vi "main.vi"() -> ()   [LabVIEW 2016]
uses:
  <vilib>/Simulation/Scripting/Companion Diagram/SimConfigNode/SimDog.xnode
  <vilib>/Simulation/Implementation/Shared/SIMSCR Execution Mode.ctl
  <vilib>/Simulation/Scripting/Companion Diagram/SimConfigNode/_simSolvers.ctl
  <vilib>/Simulation/Scripting/Companion Diagram/SimConfigNode/SimParams.ctl
  <vilib>/Simulation/Implementation/XNodeFramework/SimXNode/SimX.xnode
  <vilib>/Simulation/Model Libraries/PID/SIM PID.vi
  <vilib>/Simulation/SignalArithmetic/Implementation/NILVSim Gain.llb/SIM Gain (scalar).vi
  <vilib>/Simulation/Utility/Implementation/SIM Halt.vi
  <vilib>/Simulation/ContinuousLinear/Implementation/NILVSim Integrator new.llb/SIM Integrator (scalar).vi
  <vilib>/Simulation/ContinuousLinear/Implementation/NILVSim Transfer Function.llb/SIM Transfer Function (SISO).vi
  <vilib>/Simulation/Model Libraries/PID/SIM PID (Parallel).vi
  <vilib>/Instr/_visa.llb/VISA Configure Serial Port (Instr).vi
panel:
  in  "lower limit":dbl
  in  "upper limit":dbl
  in  "debut simulation":bool
  in  "5":bool
  in  "baud rate (9600)":u32=9600
  in  "data bits (8)":u16=8 min=5 max=8 step=1
  in  "parity (0:none)":enum16{"None", "Odd", "Even", "Mark", "Space"}(ring)
  in  "timeout (10sec)":u32=10000
  in  "VISA RESOURCE":refnum<visa-resource-name>="GPIB0::2::INSTR"
  out "Process Chart":cluster{"output":dbl, "Setpoint ":dbl}(graph)
  out "Surge Tank":dbl(slide)=49.279730305904245 scale=0.0..10.0 scale format="%.2f"
  out "Pump":bool=TRUE
  in  "PID parameters (LIC 101)":T1={"Kc"=10.0, "Ti (min)"=0.05, "Td (min)"=0.0} {"Td (min)" format="%#.6f"; "Ti (min)" format="%#.4f"; "Kc" format="%#.4f"}
  out "Flow sensor":bool
  out "Valve":bool
  out "output in limit":dbl
  out "processing output":dbl
  in  "Setpoint":dbl(knob) scale=0.0..10.0
  # "recomanded PID parameters are\nKC=0.82\nTi=0.035\nTd=0"
  # "recomanded limits\nlower limit=-0.01\nupprt limit=0.01"
  # "Marge \nd'erreur \nacceptable"
  # "Visa Configuration"
  # "LCV"
  # "101"
  # "LIC"
  # "101"
  # "LT"
  # "101"
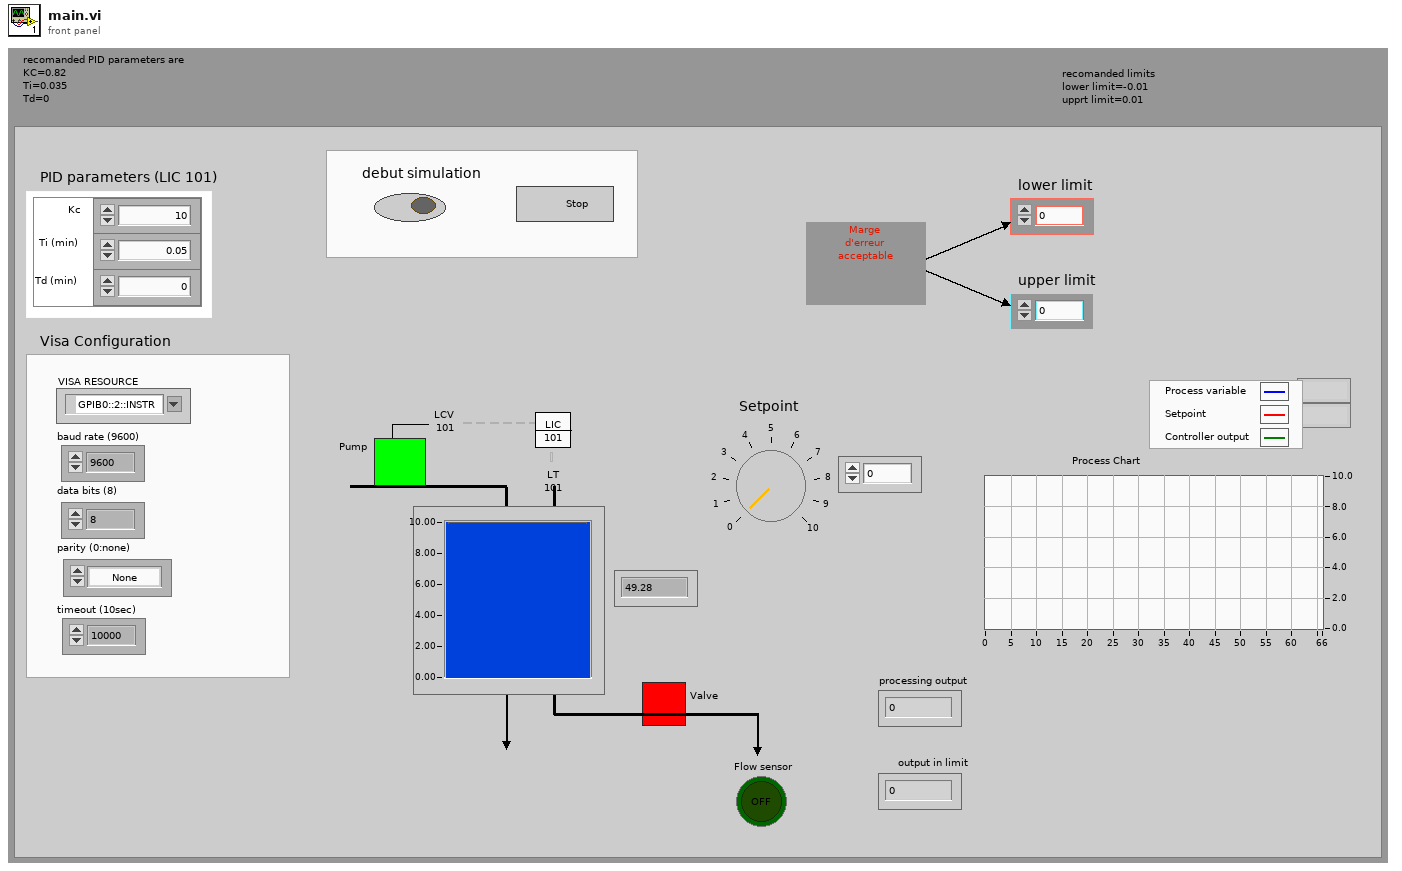
[diagram p1: front panel]
types:
  T1 = cluster{"Kc":dbl, "Ti (min)":dbl, "Td (min)":dbl}
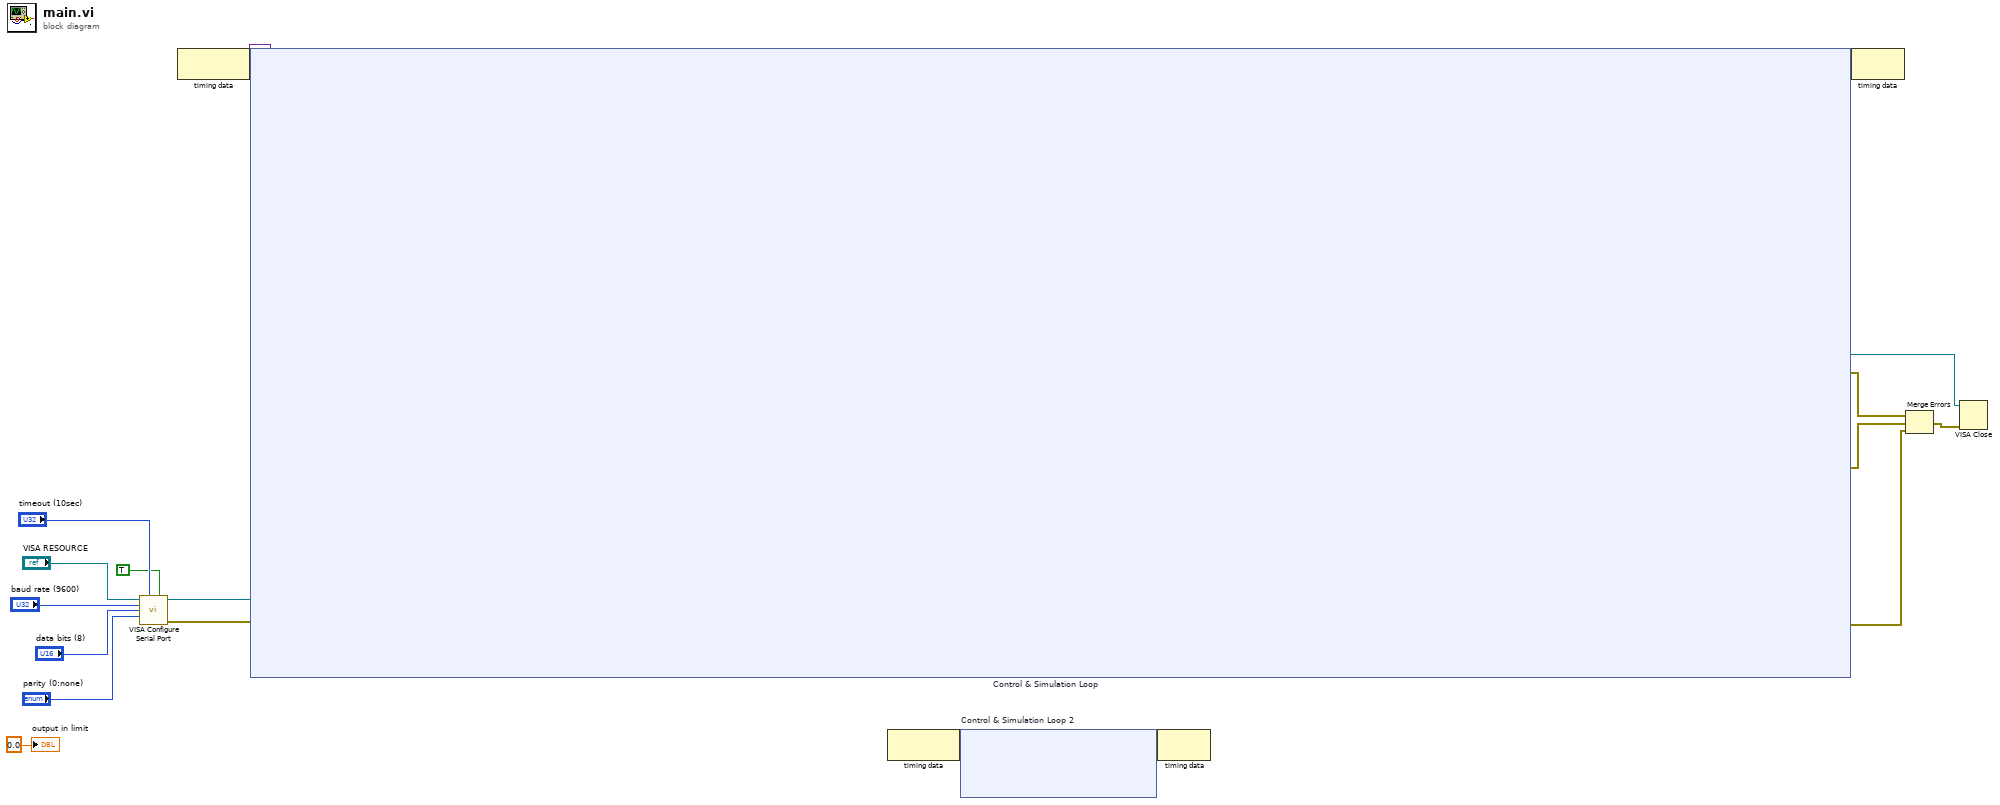
[diagram p0: block diagram]
diagram:
  n1 = call-poly "VISA Configure Serial Port"("VISA resource name"="VISA RESOURCE", "timeout (10sec)"="timeout (10sec)", "Enable Termination\nChar (T)"=TRUE ("Enable Termination\nChar (T)"), "baud rate (9600)"="baud rate (9600)", "data bits (8)"="data bits (8)", "parity (0:none)"="parity (0:none)") -> ("VISA resource name out"=w16:refnum<visa-resource-name>, "error out"=w15:errorcluster)  [unwired: 8 in]
  n2 = node-c288() -> (w18:variant)  [unwired: 1 in]
  n3 = node-c254 "Control & Simulation Loop"(w18, w16, w15) -> (w17:variant, w4:refnum<visa-resource-name>, w7:errorcluster, w6:errorcluster, w5:errorcluster)  [unwired: 2 out]
  n4 = node-c288() -> (w2:variant)  [unwired: 1 in]
  n5 = node-c254 "Control & Simulation Loop 2"(w2) -> (w1:variant)
  n6 = node-c288(w1) -> ()  [unwired: 1 out]
  n7 = node-c288(w17) -> ()  [unwired: 1 out]
  n8 = Merge Errors(w7, w6, w5) -> (w3:errorcluster)
  n9 = VISA Close(VISA resource name=w4, error in (no error)=w3) -> ()  [unwired: 1 out]
  "output in limit" <- 0.0 ("output")
